vi "st_common sub-array.vi"(9 "array 1 in":dbl[](array[numeric]), 10 "array 1 in":dbl[](array[numeric])) -> (1 "array 1 out":dbl[](array[numeric]), 2 "array 1 out":dbl[](array[numeric]), 4 "size":i32)   [LabVIEW 2024, in "NI_Gmath.lvlib"]
uses:
  NI_Gmath.lvlib
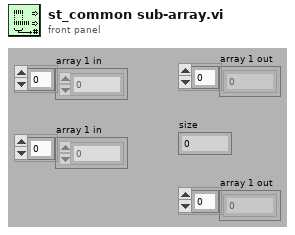
[diagram p1: front panel]
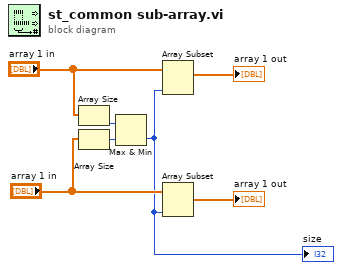
[diagram p0: block diagram]
diagram:
  n1 = Array Size(array="array 1 in") -> (size(s)=w1:i32)
  n2 = Array Size(array="array 1 in") -> (size(s)=w2:i32)
  n3 = Max & Min(x=w1, y=w2) -> (min(x,y)=w4:i32)  [unwired: 1 out]
  "size" <- w4
  n4 = Array Subset(array="array 1 in", length=w4) -> (→"array 1 out":dbl[])  [unwired: 1 in]
  n5 = Array Subset(array="array 1 in", length=w4) -> (→"array 1 out":dbl[])  [unwired: 1 in]
